vi "Example 10 - Event Bus.vi"() -> ()   [LabVIEW 2021]
uses:
  Omni-Bus/Omni_Bus.lvclass
  Event Bus/Event_Bus.lvclass
  C:/TSA/Omni-Bus/Source/Omni-Bus/Bus Access/Bus_Access.lvclass
  Local Bus/Local Bus.lvclass
  Event Bus/Support/Event Source/Polled_EventSource/Polled_EventSource.lvclass
  C:/TSA/Omni-Bus/Source/Event Bus/Support/Event Source/Event_Source.lvclass
  Local Bus/Support/Tag List Type.ctl
  <vilib>/Utility/Data Type/Type Definitions/Data Type.ctl
  <vilib>/TSA/Abstract Data Classes/Abs_Types/Type/Abs_Type.lvclass/Abs_Type.ctl
  Omni-Bus/Omni_Bus.lvclass/Omni_Bus.ctl
  Omni-Bus/Support/Write/Write DBL.vi
  Omni-Bus/Support/Read/Read DBL.vi
  Omni-Bus/Support/FindVar.vi
  <vilib>/Utility/error.llb/Clear Errors.vi
  <vilib>/TSA/Abstract Data Classes/Abs_Types/Type/Properties/Write Tag.vi
  Omni-Bus/Properties/Read Var Map.vi
  <vilib>/TSA/Abstract Data Classes/Abs_Types/Type/Properties/Read Tag.vi
  <vilib>/TSA/Abstract Data Classes/Abs_Types/Double Float/Abs_Double Float.lvclass
  C:/Program Files (x86)/National Instruments/LabVIEW 2021/vi.lib/TSA/Abstract Data Classes/Abs_Types/Type/Abs_Type.lvclass
  <vilib>/TSA/Abstract Data Classes/Abs_Types/Value/Abs_Value.lvclass
  Omni-Bus/Support/Check For Read Only Error.vi
  Omni-Bus/Support/Incorrect Tag String Error.vi
  <vilib>/TSA/Abstract Data Classes/Abs_Types/Type/Abs_Type.lvclass
  <vilib>/Utility/Data Type/NI_Data Type.lvlib
  <vilib>/ptbypt/NI_PtbyPt.lvlib
panel:
  out "Stopping":bool
  out "Waveform Chart":dbl(graph)
  out "Numeric 2":i32
  out "Numeric":i32
  in  "stop":bool
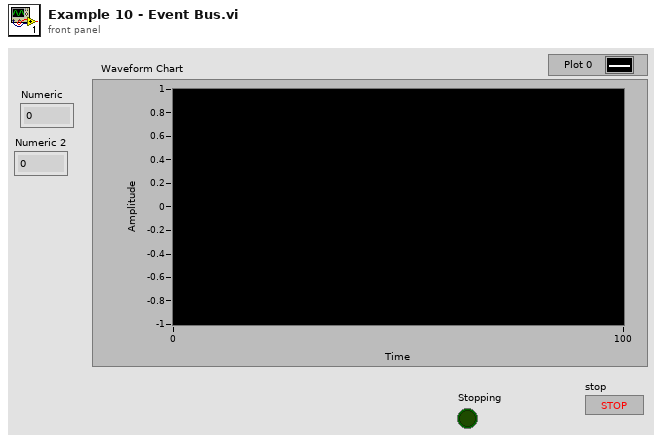
[diagram p1: front panel]
types:
  T1 = typedef "Local Bus.lvclass/Tag List Type.ctl" = cluster{"Tag":string, "Type":T2}
  T2 = typedef "NI_Data Type.lvlib/Data Type.ctl" = enum8{"Invalid Type", "Void", "I8", "I16", "I32", "I64", "U8", "U16", "U32", "U64", "Single Float", "Double Float", "Extended Float", "Single Complex", "Double Complex", "Extended Complex", "Enum U8", "Enum U16", "Enum U32", "Enum U64", "Single Float With Unit", "Double Float With Unit", "Extended Float With Unit", "Single Complex with Unit", "Double Complex with Unit", "Extended Complex with Unit", "Boolean", "String", "Path", "Picture", "Tag", "Array", "Cluster", "Variant", "LV Variant", "Waveform", "Timestamp", "Digital Waveform", "Digital Data", "ExpressData", "Refnum", "External Data", "VI", "Poly VI", "LabVIEW Class Instance", "Fixed Point", "Set Collection", "Map Collection"}
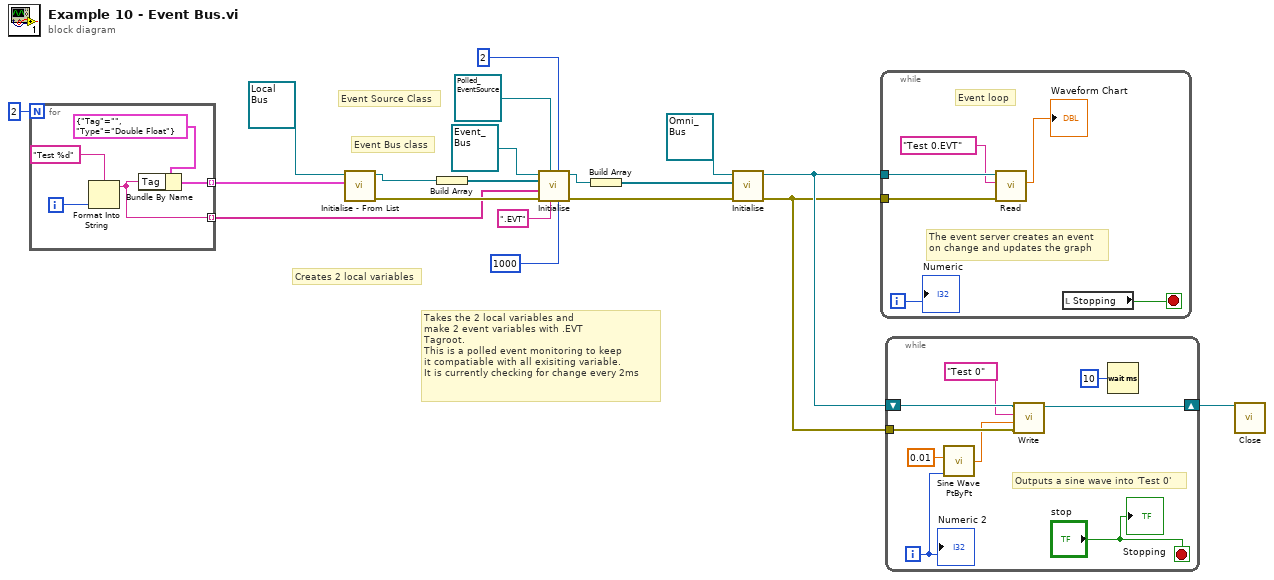
[diagram p0: block diagram]
diagram:
  # "Event Bus class"
  # "Event Source Class"
  # "Takes the 2 local variables and\nmake 2 event variables with .EVT\nTagroot.\nThis is a polled event monitoring to keep\nit compatiable with all exisiting variable.\nIt is currently checking for change every 2ms"
  # "Creates 2 local variables"
  n1 = for {
    N: 2 -> [_]
    tunnel: [w21] -> w8 mode=indexing
    tunnel: [w20] -> w5 mode=indexing
    i -> [w22]
    n2 = Format Into String(format string="Test %d", w22) -> (resulting string=w20:string)  [unwired: 2 in, 1 out]
    n3 = Bundle By Name(cluster=T1 {"Tag"="", "Type"=enum."Double Float"} ("Cluster"), "Tag"=w20) -> (w21:T1)
  }
  n4 = call "Initialise - From List.vi"("Tag List"=w8, "Local Bus in"=refnum<class "Local Bus.lvclass"> refnum) -> ("error out"=w13:errorcluster, "Local Bus out"=w12:refnum<class "Local Bus.lvclass">)  [unwired: 8 in]
  n5 = Build Array(w12) -> (w14:refnum<class "Local Bus.lvclass">[])
  n6 = call "Initialise.vi"("Default Timeout (ms)"=1000, "Poll Interval (ms)"=2, "Tag Root"=".EVT", "Event_Source.lvclass"=refnum<class "Polled_EventSource.lvclass"> refnum ("Polled_EventSource.lvclass"), "error in (no error)"=w13, "Tags to Create Events For"=w5, "Buses"=w14, "Event_Bus in"=refnum<class "Event_Bus.lvclass"> refnum) -> ("error out"=w17:errorcluster, "Event_Bus out"=w16:refnum<class "Event_Bus.lvclass">)  [unwired: 2 in]
  n7 = Build Array(w16) -> (w18:refnum<class "Event_Bus.lvclass">[])
  n8 = call-dynamic "Initialise.vi"("error in (no error)"=w17, "Bus Access"=w18, "Var Bus in"=refnum<class "Omni_Bus.lvclass"> refnum) -> ("error out"=w3:errorcluster, "Var Bus out"=w4:refnum<class "Omni_Bus.lvclass">)  [unwired: 7 in]
  n9 = while {
    tunnel: w4 -> [w30]
    tunnel: w3 -> [w29]
    i -> [w28]
    stop <- w25 stop-if-true
    # "The event server creates an event\non change and updates the graph"
    # "Event loop"
    n10 = call-poly "Read.vi"("error in (no error)"=w29, "Tag"="Test 0.EVT" ("Combo Box"), "Var Bus in"=w30) -> ("Numeric"=→"Waveform Chart":dbl)  [unwired: 6 in, 2 out]
    n11 = local read "Stopping"() -> (w25:bool)
    "Numeric" <- w28
  }
  n12 = while {
    tunnel: w3 -> [w38]
    shift-right: [w37] -> w10
    shift-left: w4 -> [w39]
    i -> [w33]
    stop <- "stop" stop-if-true
    # "Outputs a sine wave into 'Test 0'"
    n13 = call <vilib>:"Sine Wave PtByPt.vi"("time"=w33, "frequency"=0.01) -> ("sine wave"=w34:dbl)  [unwired: 2 in]
    n14 = call-poly "Write.vi"("error in (no error)"=w38, "Numeric"=w34, "Tag"="Test 0" ("Combo Box 2"), "Omni_Bus in"=w39) -> ("Omni_Bus out"=w37:refnum<class "Omni_Bus.lvclass">)  [unwired: 6 in, 1 out]
    n15 = Wait (ms)(milliseconds to wait=u32 10) -> ()  [unwired: 1 out]
    "Numeric 2" <- w33
    "Stopping" <- "stop"
  }
  n16 = call-dynamic "Close.vi"("Data in"=w10) -> ()  [unwired: 9 in, 2 out]
